vi "LidarTest.vi"(8 "error out":errorcluster, 10 "Position":cluster{"X":dbl, "Y":dbl, "Theta":dbl}) -> (0 "Error/Flow Out":errorcluster)   [LabVIEW 2018]
panel:
  out "Magnitude":dbl[](array[numeric])
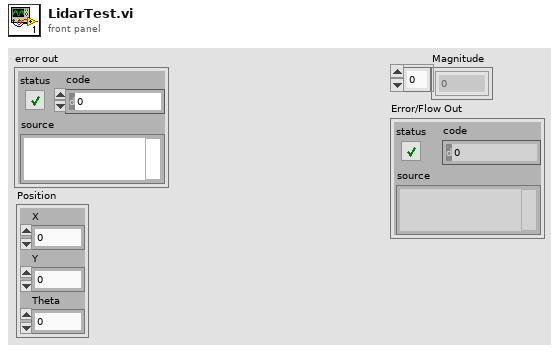
[diagram p1: front panel]
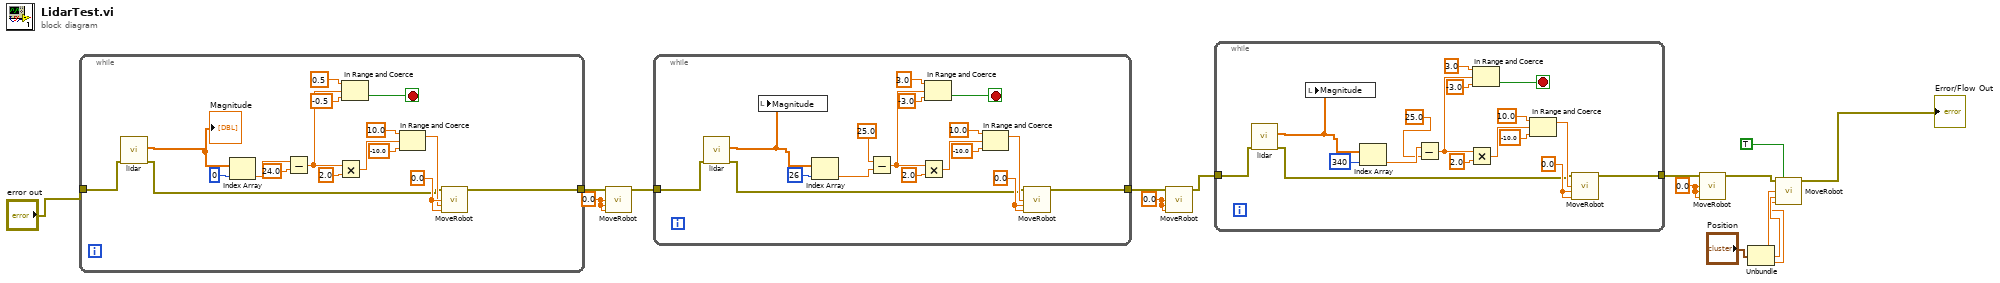
[diagram p0: block diagram]
diagram:
  w11 = 0.0 ("x (mm/s)")
  w13 = 0.0 ("x (mm/s)")
  w16 = 0.0 ("x (mm/s)")
  n1 = while {
    tunnel: "error out" -> [w18]
    tunnel: [w27] -> w15
    stop <- w30 stop-if-true
    w24 = 0.0 ("x (mm/s)")
    n2 = call "lidar.vi"("error in (no error)"=w18) -> ("error out"=w17:errorcluster, "range Out"=w19:dbl[])  [unwired: 8 in, 1 out]
    "Magnitude" <- w19
    n3 = Index Array(array=w19, index=0) -> (element=w32:dbl)
    n4 = Subtract(x=w32, y=24.0) -> (x-y=w26:dbl)
    n5 = Multiply(x=w26, y=2.0) -> (x*y=w22:dbl)
    n6 = In Range and Coerce(upper limit=0.5, x=w26, lower limit=-0.5) -> (In Range?=w30:bool)  [unwired: 1 out]
    n7 = In Range and Coerce(upper limit=10.0, x=w22, lower limit=-10.0) -> (coerced(x)=w23:dbl)  [unwired: 1 out]
    n8 = call "MoveRobot.vi"("Error/Flow In"=w17, "x (mm/s)"=w24, "y (mm/s)"=w23, "theta (rad/s)"=w24) -> ("Error/Flow Out"=w27:errorcluster)  [unwired: 10 in, 1 out]
  }
  n9 = call "MoveRobot.vi"("Error/Flow In"=w15, "x (mm/s)"=w16, "y (mm/s)"=w16, "theta (rad/s)"=w16) -> ("Error/Flow Out"=w12:errorcluster)  [unwired: 10 in, 1 out]
  n10 = while {
    tunnel: w12 -> [w35]
    tunnel: [w46] -> w14
    stop <- w49 stop-if-true
    w38 = 0.0 ("x (mm/s)")
    n11 = call "lidar.vi"("error in (no error)"=w35) -> ("error out"=w34:errorcluster, "range Out"=w40:dbl[])  [unwired: 8 in, 1 out]
    n12 = local write "Magnitude"(w40) -> ()
    n13 = Index Array(array=w40, index=26) -> (element=w36:dbl)
    n14 = Subtract(x=25.0 ("y"), y=w36) -> (x-y=w45:dbl)
    n15 = Multiply(x=w45, y=2.0) -> (x*y=w43:dbl)
    n16 = In Range and Coerce(upper limit=3.0, x=w45, lower limit=-3.0) -> (In Range?=w49:bool)  [unwired: 1 out]
    n17 = In Range and Coerce(upper limit=10.0, x=w43, lower limit=-10.0) -> (coerced(x)=w39:dbl)  [unwired: 1 out]
    n18 = call "MoveRobot.vi"("Error/Flow In"=w34, "x (mm/s)"=w39, "y (mm/s)"=w38, "theta (rad/s)"=w38) -> ("Error/Flow Out"=w46:errorcluster)  [unwired: 10 in, 1 out]
  }
  n19 = call "MoveRobot.vi"("Error/Flow In"=w14, "x (mm/s)"=w13, "y (mm/s)"=w13, "theta (rad/s)"=w13) -> ("Error/Flow Out"=w9:errorcluster)  [unwired: 10 in, 1 out]
  n20 = while {
    tunnel: w9 -> [w52]
    tunnel: [w63] -> w10
    stop <- w66 stop-if-true
    w55 = 0.0 ("x (mm/s)")
    n21 = call "lidar.vi"("error in (no error)"=w52) -> ("error out"=w51:errorcluster, "range Out"=w57:dbl[])  [unwired: 8 in, 1 out]
    n22 = local write "Magnitude"(w57) -> ()
    n23 = Index Array(array=w57, index=340) -> (element=w54:dbl)
    n24 = Subtract(x=w54, y=25.0) -> (x-y=w62:dbl)
    n25 = Multiply(x=w62, y=2.0) -> (x*y=w60:dbl)
    n26 = In Range and Coerce(upper limit=3.0, x=w62, lower limit=-3.0) -> (In Range?=w66:bool)  [unwired: 1 out]
    n27 = In Range and Coerce(upper limit=10.0, x=w60, lower limit=-10.0) -> (coerced(x)=w56:dbl)  [unwired: 1 out]
    n28 = call "MoveRobot.vi"("Error/Flow In"=w51, "x (mm/s)"=w56, "y (mm/s)"=w55, "theta (rad/s)"=w55) -> ("Error/Flow Out"=w63:errorcluster)  [unwired: 10 in, 1 out]
  }
  n29 = call "MoveRobot.vi"("Error/Flow In"=w10, "x (mm/s)"=w11, "y (mm/s)"=w11, "theta (rad/s)"=w11) -> ("Error/Flow Out"=w7:errorcluster)  [unwired: 10 in, 1 out]
  n30 = Unbundle("Position") -> ("X"=w3:dbl, "Y"=w2:dbl, "Theta"=w1:dbl)
  n31 = call "MoveRobot.vi"("Error/Flow In"=w7, "Reset"=TRUE, "x (mm/s)"=w3, "y (mm/s)"=w2, "theta (rad/s)"=w1) -> ("Error/Flow Out"=→"Error/Flow Out":errorcluster)  [unwired: 9 in, 1 out]
